vi "EditableMenu.vi"() -> ()   [LabVIEW 2020]
uses:
  <vilib>/Utility/miscctls.llb/LVMenuShortCut.ctl
panel:
  in  "stop":bool
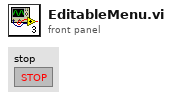
[diagram p1: front panel]
types:
  T1 = typedef "LVMenuShortCut.ctl" = cluster{"Include Shift Key?":bool, "Include Ctrl Key?":bool, "Shortcut Key":string}
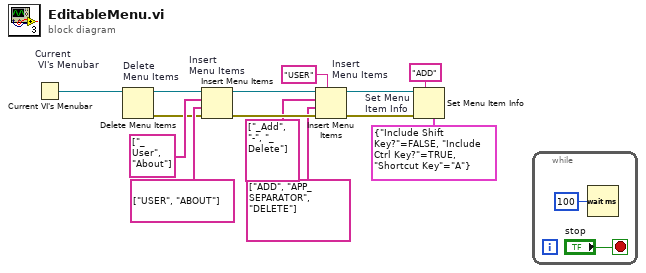
[diagram p0: block diagram]
diagram:
  n1 = Current VI's Menubar "Current\n VI's Menubar"() -> (w13:refnum<k9>)
  n2 = Delete Menu Items "Delete\nMenu Items"(9:w13) -> (0:w10:errorcluster, 3:w14:refnum<k9>)  [unwired: 3 in]
  n3 = Insert Menu Items "Insert\nMenu Items"(6:w10, 7:string[] ["USER", "ABOUT"] ("item tags"), 8:string[] ["_User", "About"] ("item names"), 9:w14) -> (0:w7:errorcluster, 3:w6:refnum<k9>)  [unwired: 2 in, 1 out]
  n4 = Insert Menu Items "Insert\nMenu Items"(5:"USER" ("menu tag"), 6:w7, 7:string[] ["ADD", "APP_SEPARATOR", "DELETE"] ("item tags"), 8:string[] ["_Add", "-", "_Delete"] ("item names"), 9:w6) -> (0:w4:errorcluster, 3:w5:refnum<k9>)  [unwired: 1 in, 1 out]
  n5 = Set Menu Item Info "Set Menu\nItem Info"(4:T1 {"Include Shift Key?"=FALSE, "Include Ctrl Key?"=TRUE, "Shortcut Key"="A"} ("short cut"), 7:"ADD" ("item tag"), 8:w4, 11:w5) -> ()  [unwired: 3 in, 2 out]
  n6 = while {
    stop <- "stop" stop-if-true
    n7 = Wait (ms)(milliseconds to wait=u32 100) -> ()  [unwired: 1 out]
  }
